vi "Delete Temp Files.vi"(8 "error in":errorcluster) -> (0 "error out":errorcluster)   [LabVIEW 2012]
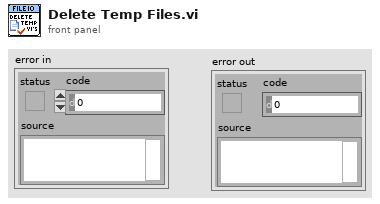
[diagram p1: front panel]
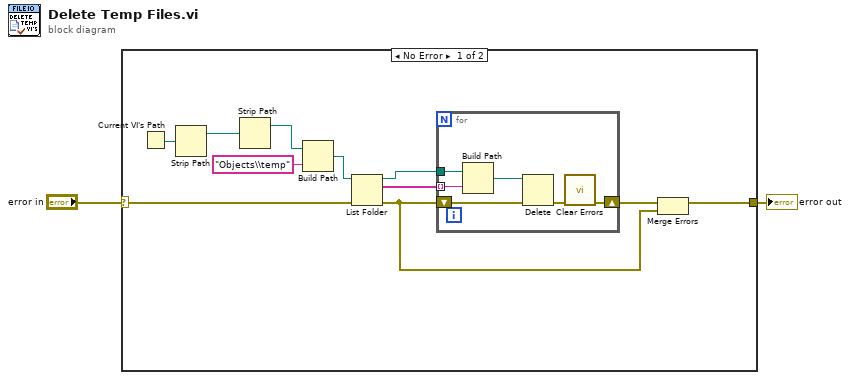
[diagram p0: block diagram]
diagram:
  n1 = case shown="No Error" "error in" {
    selector: "error in" -> [w3 w20]
    tunnel: [w4 w20] -> w1
    frame No Error {
      n2 = Current VI's Path() -> (path=w11:path)
      n3 = Strip Path(path=w11) -> (stripped path=w10:path)  [unwired: 1 out]
      n4 = Strip Path(path=w10) -> (stripped path=w13:path)  [unwired: 1 out]
      n5 = Build Path(base path=w13, name or relative path="Objects\\temp") -> (appended path=w9:path)
      n6 = List Folder(path=w9, error in=w3) -> (path out=w7:path, filenames=w8:string[], error out=w5:errorcluster)  [unwired: 2 in, 1 out]
      n7 = for {
        tunnel: w8 -> [w19] mode=indexing
        tunnel: w7 -> [w18]
        shift-right: [w15] -> w6
        shift-left: w5 -> [w14]
        n8 = Build Path(base path=w18, name or relative path=w19) -> (appended path=w17:path)
        n9 = Delete(path (use dialog)=w17, error in=w14) -> (error out=w16:errorcluster)  [unwired: 3 in, 2 out]
        n10 = call <vilib>:"Clear Errors.vi"("error in (no error)"=w16) -> ("error out"=w15:errorcluster)  [unwired: 6 in]
      }
      n11 = Merge Errors(w6, w5) -> (w4:errorcluster)
    }
    frame Error {
    }
  }
  "error out" <- w1
